vi "calculate_phi_p.vi"(7 "phi":dbl, 8 "Error In":errorcluster, 9 "p_hat_parallel":dbl[](array[numeric]), 10 "p_hat_perpendicular":dbl[](array[numeric]), 11 "c_hat":dbl[](array[numeric])) -> (0 "Error Out":errorcluster, 2 "phi_p_2":dbl, 3 "phi_p_1":dbl)   [LabVIEW 2019]
doc: "Calculate phi from formula 4 in Wilen(2000). All inputs and outputs are in degrees."
panel:
  out "output variable 2":dbl
  out "output variable":dbl
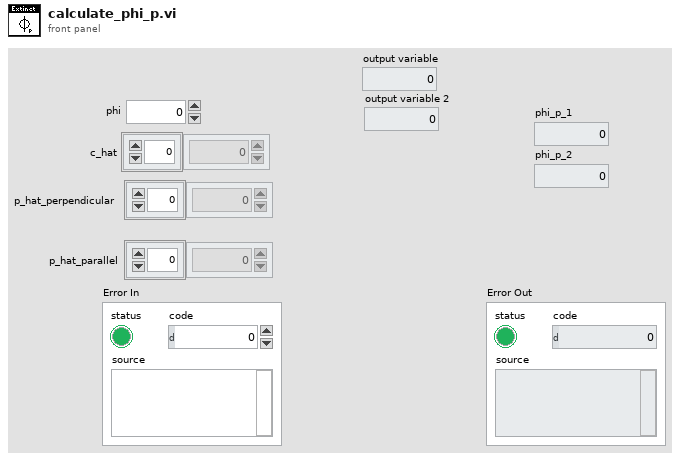
[diagram p1: front panel]
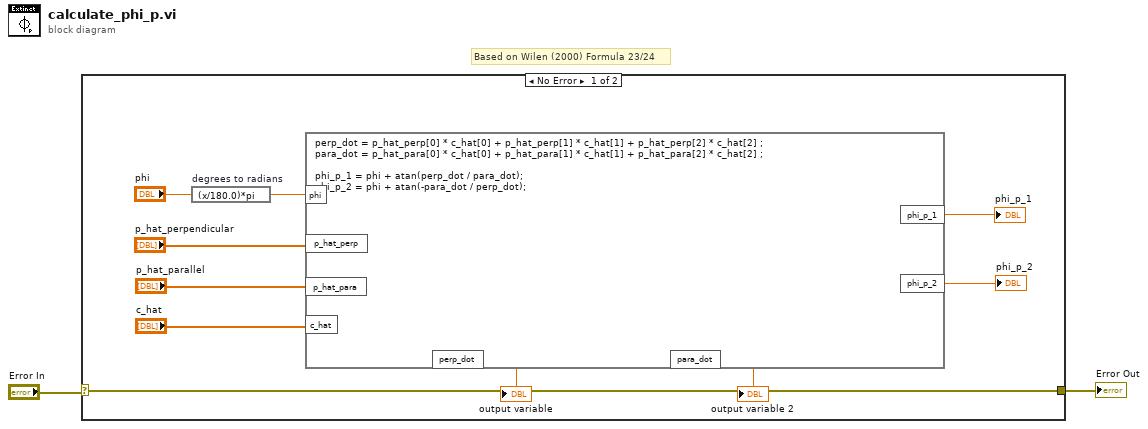
[diagram p0: block diagram]
diagram:
  # "Based on Wilen (2000) Formula 23/24"
  n1 = case shown="No Error" "Error In" {
    selector: "Error In" -> [w12 w13]
    tunnel: [w12 w13] -> w1
    frame No Error {
      n2 = expression code="(x/180.0)*pi" "degrees to radians"("phi") -> (w11:dbl)
      n3 = formula code="perp_dot = p_hat_perp[0] * c_hat[0] + p_hat_perp[1] * c_hat[1] + p_hat_perp[2] * c_hat[2] ;\npara_dot = p_hat_para[0] * c_hat[0] + p_hat_para[1] * c_hat[1] + p_hat_para[2] * c_hat[2] ;\n\nphi_p_1 = phi + atan(perp_dot / para_dot);\nphi_p_2 = phi + atan(-para_dot / perp_dot);"("phi"=w11, "p_hat_perp"="p_hat_perpendicular", "p_hat_para"="p_hat_parallel", "c_hat"="c_hat") -> ("phi_p_1"=→"phi_p_1":dbl, "phi_p_2"=→"phi_p_2":dbl, "perp_dot"=→"output variable":dbl, "para_dot"=→"output variable 2":dbl)
    }
    frame Error {
    }
  }
  "Error Out" <- w1
